vi "checkLBValue2.vi"() -> (0 "LB new status":bool[](array[boolean]))   [LabVIEW 2012]
uses:
  <vilib>/Instr/_visa.llb/Select Event Type.ctl
  GlobalArduino.vi
  GlobalLB.vi
panel:
  out "error out":errorcluster
  out "Break Detected?":bool
  out "Timeout?":bool
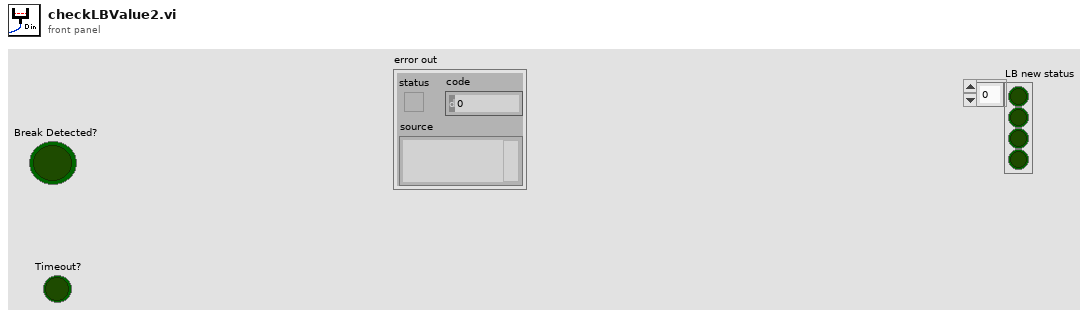
[diagram p1: front panel]
types:
  T1 = typedef "Select Event Type.ctl" = u32
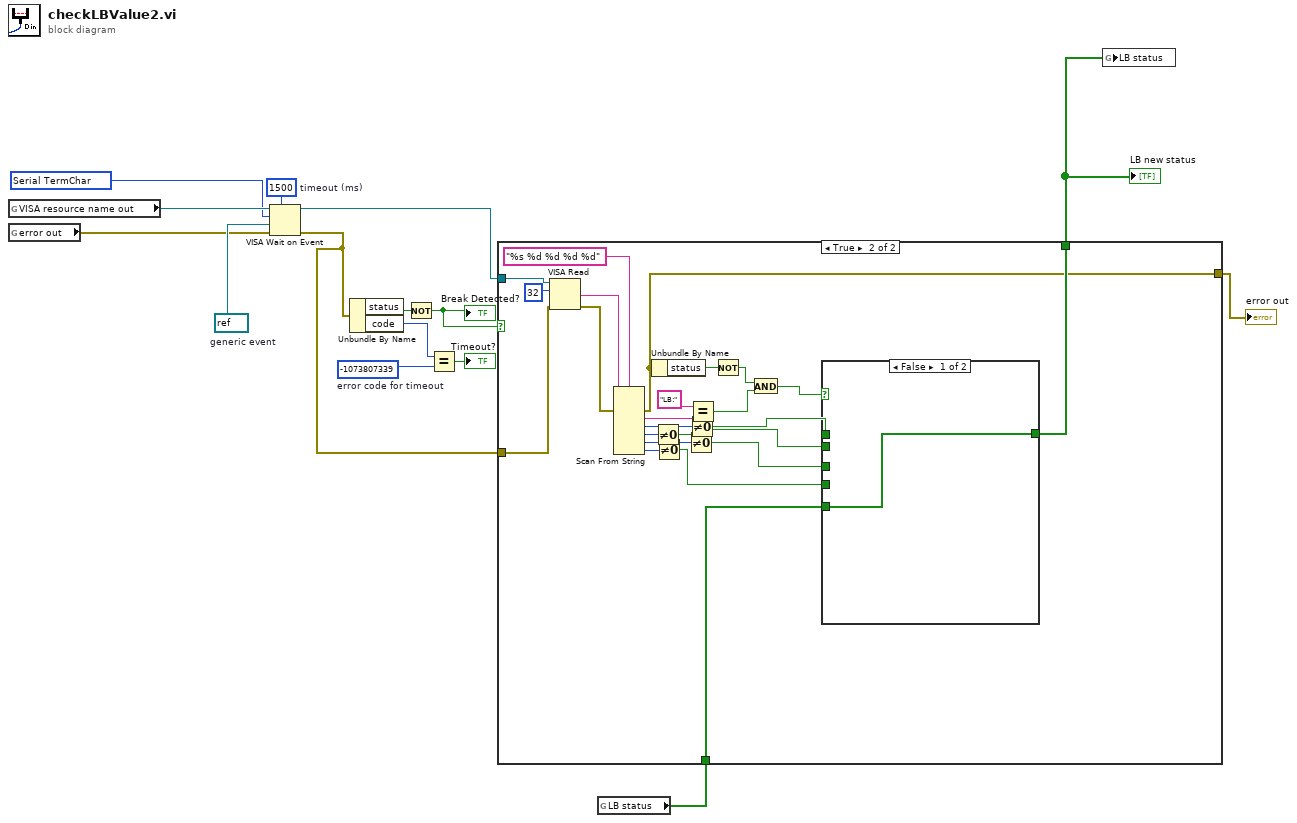
[diagram p0: block diagram]
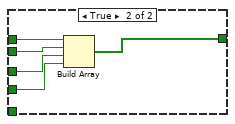
[diagram p3: hidden frame]
diagram:
  w7 = T1 1073684516 items=["Service Request"=1073684491, "Trigger"=3221168138, "Clear"=1073684493, "VXI Signal"=1073684512, "VXI/VME Interrupt"=3221168161, "VXI/VME Sysfail"=1073684509, "VXI/VME Sysreset"=1073684510, "GPIB CIC"=1073684498, "GPIB Talk"=1073684499, "GPIB Listen"=1073684500, "PXI Interrupt"=1073684514, "Serial Break"=1073684515, "Serial TermChar"=1073684516, "Serial CTS"=1073684521, "Serial DSR"=1073684522, "Serial DCD"=1073684524, "Serial RI"=1073684526, "Serial Character"=1073684533, "USB Interrupt"=1073684535, "All Enabled"=1073709055] ("Event Type")
  w9 = refnum<visa-resource-name> refnum  # generic event
  w13 = -1073807339  # error code for timeout
  w15 = u32 1500  # timeout (ms)
  n1 = global read "GlobalArduino.vi" "VISA resource name out"() -> (w8:refnum<visa-resource-name>)
  n2 = global read "GlobalArduino.vi" "error out"() -> (w6:errorcluster)
  n3 = VISA Wait on Event(7:w15, 8:w6, 9:w9, 10:w7, 11:w8) -> (0:w3:errorcluster, 3:w1:refnum<visa-resource-name>)  [unwired: 2 out]
  n4 = Unbundle By Name(w3) -> ("status"=w12:bool, "code"=w14:i32)
  n5 = Not(x=w12) -> (.not. x?=w10:bool)
  "Break Detected?" <- w10
  n6 = Equal?(x=w14, y=w13) -> (x = y?=→"Timeout?":bool)
  n7 = global read "GlobalLB.vi" "LB status"() -> (w5:bool[])
  n8 = case shown="True" w10 {
    tunnel: w5 -> [w17 w22]
    tunnel: [w17 w21] -> w4
    tunnel: w3 -> [w16 w19]
    tunnel: [w16 w18] -> w2
    tunnel: w1 -> [_ w20]
    frame False {
    }
    frame True {
      n9 = VISA Read(VISA resource name=w20, byte count=u32 32, error in (no error)=w19) -> (read buffer=w39:string, error out=w23:errorcluster)  [unwired: 2 out]
      n10 = Scan From String(format string="%s %d %d %d %d", input string=w39, error in=w23) -> (error out=w18:errorcluster, output 1=w37:string, output 2=w35:i32, output 3=w34:i32, output 4=w29:i32, output 5=w28:i32)  [unwired: 6 in, 2 out]
      n11 = Unbundle By Name(w18) -> ("status"=w33:bool)
      n12 = Not Equal To 0?(x=w34) -> (x != 0?=w26:bool)
      n13 = Not Equal To 0?(x=w28) -> (x != 0?=w24:bool)
      n14 = Not Equal To 0?(x=w29) -> (x != 0?=w25:bool)
      n15 = Not Equal To 0?(x=w35) -> (x != 0?=w27:bool)
      n16 = Equal?(x="LB:", y=w37) -> (x = y?=w31:bool)
      n17 = Not(x=w33) -> (.not. x?=w32:bool)
      n18 = And(x=w32, y=w31) -> (x .and. y?=w30:bool)
      n19 = case shown="False" w30 {
        tunnel: [w41 w42] -> w21
        tunnel: w22 -> [w41 _]
        tunnel: w27 -> [_ w46]
        tunnel: w26 -> [_ w45]
        tunnel: w25 -> [_ w44]
        tunnel: w24 -> [_ w43]
        frame False {
        }
        frame True {
          n20 = Build Array(w46, w45, w44, w43) -> (w42:bool[])
        }
      }
    }
  }
  "LB new status" <- w4
  "error out" <- w2
  n21 = global write "GlobalLB.vi" "LB status"(w4) -> ()
